vi "Generic command handler.vi"(8 "error in (no error)":errorcluster, 10 "Message in":refnum<class "GenericMessage.lvclass">, 11 "StageSPIM in":refnum<class "StageSPIM.lvclass">) -> (0 "error out":errorcluster, 2 "value":string, 3 "StageSPIM out":refnum<class "StageSPIM.lvclass">)   [LabVIEW 2012, in "StageSPIM.lvclass"]
doc: "The generic_command_handler processes the command 'generic'. Commands which are not part of the predefined list of commands fall under the 'generic' command for special activity."
uses:
  StageSPIM.lvclass
  <vilib>/Distrio/Murmex/GenericMessage/GenericMessage.lvclass
  <vilib>/Distrio/Murmex/Murmex/Murmex.lvclass
  StageSPIM.lvclass/StageSPIM.ctl
  <vilib>/Distrio/Murmex/ProceedMessage/ProceedMessage.lvclass
  <vilib>/Distrio/Murmex/Message/Message.lvclass
panel:
  # "This method is called when the GENERIC\ntrigger is sent. \n\nOverride this method when your component needs to\nrespond to this trigger. \n\nCall parent for proper implementation"
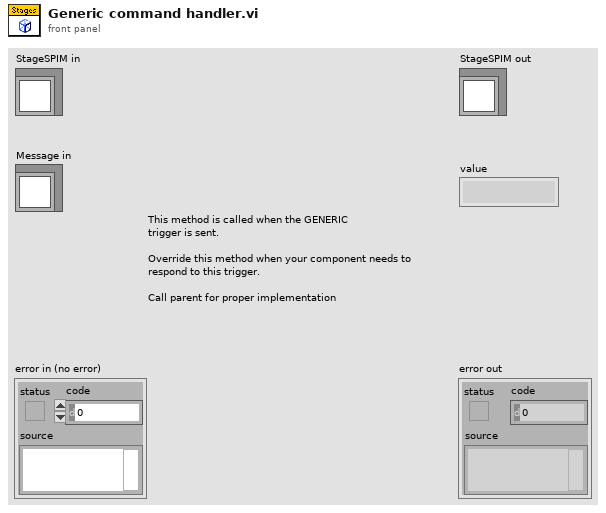
[diagram p1: front panel]
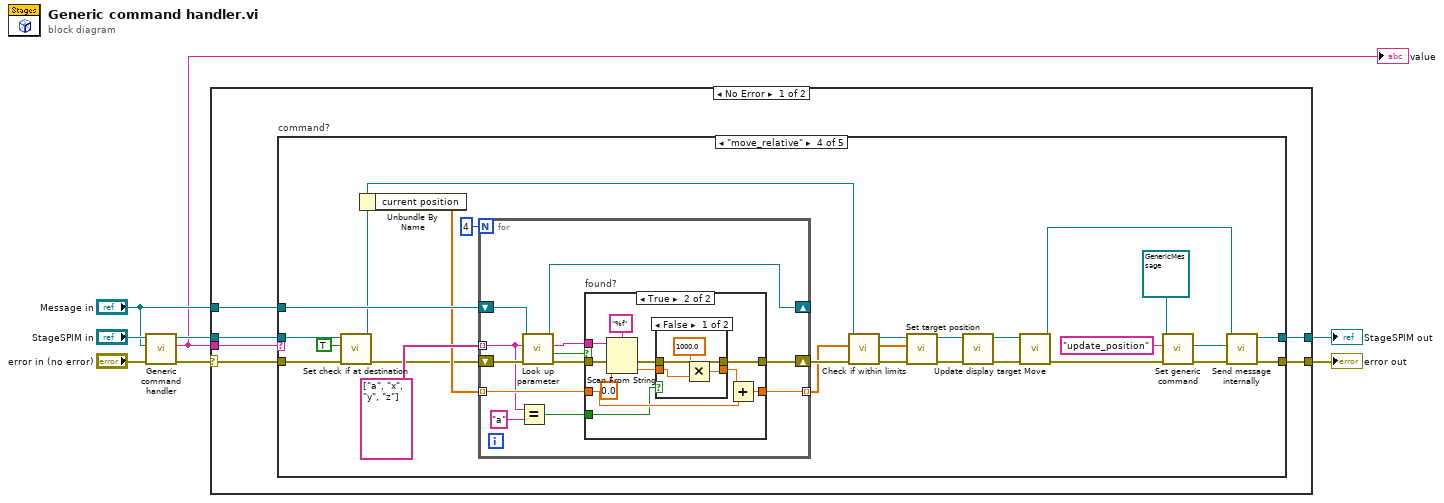
[diagram p0: block diagram]
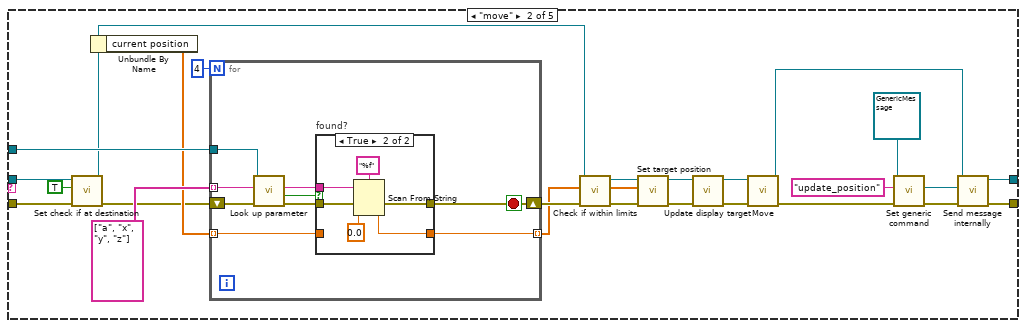
[diagram p3: hidden frame]
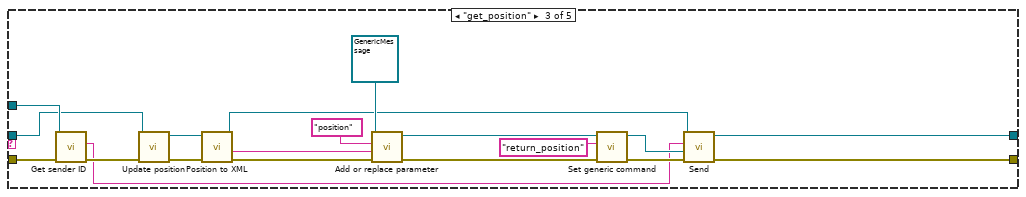
[diagram p5: hidden frame]
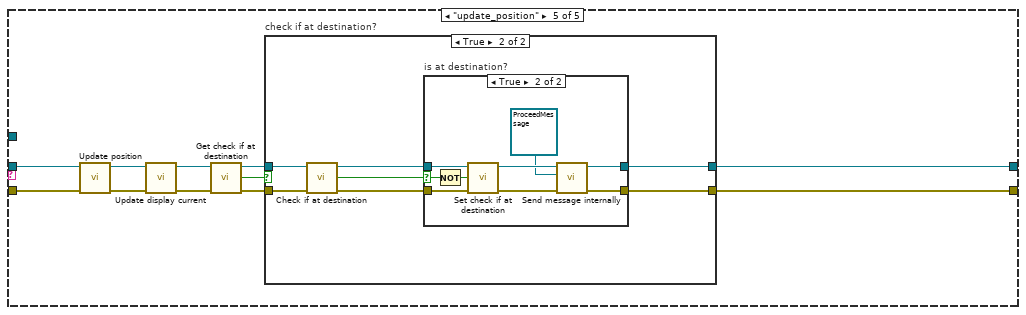
[diagram p8: hidden frame]
diagram:
  n1 = call-parent "Generic command handler.vi"("error in (no error)"="error in (no error)", "Message in"="Message in", "Murmex in"="StageSPIM in") -> ("error out"=w6:errorcluster, "value"=w3:string, "Murmex out"=w5:refnum<class "StageSPIM.lvclass">)  [unwired: 6 in]
  "value" <- w3
  n2 = case shown="No Error" w6 {
    selector: w6 -> [w13 w167]
    tunnel: w3 -> [w14 _]
    tunnel: w5 -> [w12 w168]
    tunnel: "Message in" -> [w11 _]
    tunnel: [w10 w167] -> w2
    tunnel: [w9 w168] -> w1
    frame No Error {
      n3 = case "command?" shown="\"move_relative\"" w14 {
        tunnel: w13 -> [w15 w31 w78 w93 w146]
        tunnel: w12 -> [w16 w33 w64 w95 w145]
        tunnel: w11 -> [_ w38 w77 w100 _]
        tunnel: [w15 w24 w60 w86 w140] -> w10
        tunnel: [w16 w21 w61 w83 w141] -> w9
        frame Default {
        }
        frame "move" {
          n4 = call-dynamic "Set check if at destination.vi"("error in (no error)"=w31, "check if at destination"=TRUE, "StageSPIM in"=w33) -> ("error out"=w30:errorcluster, "StageSPIM out"=w32:refnum<class "StageSPIM.lvclass">)  [unwired: 7 in]
          n5 = Unbundle By Name(w32) -> ("current position"=w35:dbl[])
          n6 = for {
            N: 4 -> [_]
            shift-right: [w43] -> w39
            shift-left: w30 -> [w51]
            tunnel: string[] ["a", "x", "y", "z"] -> [w50] mode=indexing
            tunnel: w35 -> [w45] mode=indexing
            tunnel: [w44] -> w34 mode=indexing
            tunnel: w38 -> [w46]
            stop <- w43 stop-if-true
            n7 = call <vilib>:"Look up parameter.vi"("error in (no error)"=w51, "name"=w50, "Message in"=w46) -> ("error out"=w49:errorcluster, "found?"=w48:bool, "key"=w47:string)  [unwired: 5 in, 1 out]
            n8 = case "found?" shown="True" w48 {
              tunnel: w49 -> [w53 w59]
              tunnel: [w53 w58] -> w43
              tunnel: w47 -> [_ w56]
              tunnel: [w52 w54] -> w44
              tunnel: w45 -> [w52 _]
              frame False {
              }
              frame True {
                n9 = Scan From String(format string="%f", input string=w56, error in=w59, default 1=0.0 ("default value 1")) -> (error out=w58:errorcluster, output 1=w54:dbl)  [unwired: 1 in, 2 out]
              }
            }
          }
          n10 = call-dynamic "Check if within limits.vi"("error in (no error)"=w39, "Position array in"=w34, "StageSPIM in"=w32) -> ("error out"=w41:errorcluster, "Approved postion array"=w40:dbl[], "StageSPIM out"=w42:refnum<class "StageSPIM.lvclass">)  [unwired: 4 in, 2 out]
          n11 = call-dynamic "Set target position.vi"("error in (no error)"=w41, "target position"=w40, "StageSPIM in"=w42) -> ("error out"=w20:errorcluster, "StageSPIM out"=w18:refnum<class "StageSPIM.lvclass">)  [unwired: 7 in]
          n12 = call-dynamic "Update display target.vi"("error in (no error)"=w20, "StageSPIM in"=w18) -> ("error out"=w19:errorcluster, "StageSPIM out"=w17:refnum<class "StageSPIM.lvclass">)  [unwired: 8 in]
          n13 = call-dynamic "Move.vi"("error in (no error)"=w19, "StageSPIM in"=w17) -> ("error out"=w28:errorcluster, "StageSPIM out"=w22:refnum<class "StageSPIM.lvclass">)  [unwired: 8 in]
          n14 = call <vilib>:"Set generic command.vi"("error in (no error)"=w28, "generic command"="update_position", "GenericMessage in"=refnum<class "GenericMessage.lvclass"> refnum ("Distrio Murmex 1.1:GenericMessage")) -> ("error out"=w27:errorcluster, "GenericMessage out"=w23:refnum<class "GenericMessage.lvclass">)  [unwired: 7 in]
          n15 = call <vilib>:"Send message internally.vi"("error in (no error)"=w27, "Message"=w23, "Murmex in"=w22) -> ("error out"=w24:errorcluster, "Murmex out"=w21:refnum<class "StageSPIM.lvclass">)  [unwired: 7 in]
        }
        frame "get_position" {
          n16 = call <vilib>:"Get sender ID.vi"("error in (no error)"=w78, "Message in"=w77) -> ("error out"=w76:errorcluster, "sender"=w72:string)  [unwired: 7 in, 1 out]
          n17 = call-dynamic "Update position.vi"("error in (no error)"=w76, "StageSPIM in"=w64) -> ("error out"=w66:errorcluster, "StageSPIM out"=w63:refnum<class "StageSPIM.lvclass">)  [unwired: 8 in]
          n18 = call-dynamic "Position to XML.vi"("error in (no error)"=w66, "StageSPIM in"=w63) -> ("error out"=w65:errorcluster, "XML string"=w62:string, "StageSPIM out"=w67:refnum<class "StageSPIM.lvclass">)  [unwired: 7 in]
          n19 = call <vilib>:"Add or replace parameter.vi"("error in (no error)"=w65, "value"=w62, "name"="position", "Message in"=refnum<class "GenericMessage.lvclass"> refnum ("Distrio Murmex 1.1:GenericMessage")) -> ("error out"=w70:errorcluster, "Message out"=w69:refnum<class "GenericMessage.lvclass">)  [unwired: 6 in]
          n20 = call <vilib>:"Set generic command.vi"("error in (no error)"=w70, "generic command"="return_position", "GenericMessage in"=w69) -> ("error out"=w74:errorcluster, "GenericMessage out"=w73:refnum<class "GenericMessage.lvclass">)  [unwired: 7 in]
          n21 = call <vilib>:"Send.vi"("error in (no error)"=w74, "Message"=w73, "recipient"=w72, "Murmex in"=w67) -> ("error out"=w60:errorcluster, "Murmex out"=w61:refnum<class "StageSPIM.lvclass">)  [unwired: 6 in]
        }
        frame "move_relative" {
          n22 = call-dynamic "Set check if at destination.vi"("error in (no error)"=w93, "check if at destination"=TRUE, "StageSPIM in"=w95) -> ("error out"=w92:errorcluster, "StageSPIM out"=w94:refnum<class "StageSPIM.lvclass">)  [unwired: 7 in]
          n23 = Unbundle By Name(w94) -> ("current position"=w97:dbl[])
          n24 = for {
            N: 4 -> [_]
            shift-right: [w113] -> w101
            shift-left: w92 -> [w116]
            tunnel: string[] ["a", "x", "y", "z"] -> [w107] mode=indexing
            shift-right: [w110] -> _
            shift-left: w100 -> [w111]
            tunnel: w97 -> [w109] mode=indexing
            tunnel: [w108] -> w96 mode=indexing
            n25 = Equal?(x=w107, y="a") -> (x = y?=w105:bool)
            n26 = call <vilib>:"Look up parameter.vi"("error in (no error)"=w116, "name"=w107, "Message in"=w111) -> ("error out"=w115:errorcluster, "found?"=w114:bool, "key"=w112:string, "Message out"=w110:refnum<class "GenericMessage.lvclass">)  [unwired: 5 in]
            n27 = case "found?" shown="True" w114 {
              tunnel: w115 -> [w118 w129]
              tunnel: [w118 w122] -> w113
              tunnel: w112 -> [_ w127]
              tunnel: [w117 w125] -> w108
              tunnel: w109 -> [w117 w124]
              tunnel: w105 -> [_ w123]
              frame False {
              }
              frame True {
                n28 = Scan From String(format string="%f", input string=w127, error in=w129, default 1=0.0 ("default value 1")) -> (error out=w121:errorcluster, output 1=w119:dbl)  [unwired: 1 in, 2 out]
                n29 = case shown="False" w123 {
                  tunnel: [w133 w135] -> w122
                  tunnel: w121 -> [w133 w135]
                  tunnel: [w132 w134] -> w120
                  tunnel: w119 -> [w131 w134]
                  frame False {
                    n30 = Multiply(x=1000.0, y=w131) -> (x*y=w132:dbl)
                  }
                  frame True {
                  }
                }
                n31 = Add(x=w120, y=w124) -> (x+y=w125:dbl)
              }
            }
          }
          n32 = call-dynamic "Check if within limits.vi"("error in (no error)"=w101, "Position array in"=w96, "StageSPIM in"=w94) -> ("error out"=w103:errorcluster, "Approved postion array"=w102:dbl[], "StageSPIM out"=w104:refnum<class "StageSPIM.lvclass">)  [unwired: 4 in, 2 out]
          n33 = call-dynamic "Set target position.vi"("error in (no error)"=w103, "target position"=w102, "StageSPIM in"=w104) -> ("error out"=w82:errorcluster, "StageSPIM out"=w79:refnum<class "StageSPIM.lvclass">)  [unwired: 7 in]
          n34 = call-dynamic "Update display target.vi"("error in (no error)"=w82, "StageSPIM in"=w79) -> ("error out"=w81:errorcluster, "StageSPIM out"=w80:refnum<class "StageSPIM.lvclass">)  [unwired: 8 in]
          n35 = call-dynamic "Move.vi"("error in (no error)"=w81, "StageSPIM in"=w80) -> ("error out"=w90:errorcluster, "StageSPIM out"=w84:refnum<class "StageSPIM.lvclass">)  [unwired: 8 in]
          n36 = call <vilib>:"Set generic command.vi"("error in (no error)"=w90, "generic command"="update_position", "GenericMessage in"=refnum<class "GenericMessage.lvclass"> refnum ("Distrio Murmex 1.1:GenericMessage")) -> ("error out"=w89:errorcluster, "GenericMessage out"=w85:refnum<class "GenericMessage.lvclass">)  [unwired: 7 in]
          n37 = call <vilib>:"Send message internally.vi"("error in (no error)"=w89, "Message"=w85, "Murmex in"=w84) -> ("error out"=w86:errorcluster, "Murmex out"=w83:refnum<class "StageSPIM.lvclass">)  [unwired: 7 in]
        }
        frame "update_position" {
          n38 = call-dynamic "Update position.vi"("error in (no error)"=w146, "StageSPIM in"=w145) -> ("error out"=w139:errorcluster, "StageSPIM out"=w137:refnum<class "StageSPIM.lvclass">)  [unwired: 8 in]
          n39 = call-dynamic "Update display current.vi"("error in (no error)"=w139, "StageSPIM in"=w137) -> ("error out"=w138:errorcluster, "StageSPIM out"=w136:refnum<class "StageSPIM.lvclass">)  [unwired: 8 in]
          n40 = call-dynamic "Get check if at destination.vi"("error in (no error)"=w138, "StageSPIM in"=w136) -> ("error out"=w143:errorcluster, "check if at destination"=w144:bool, "StageSPIM out"=w142:refnum<class "StageSPIM.lvclass">)  [unwired: 7 in]
          n41 = case "check if at destination?" shown="True" w144 {
            tunnel: w143 -> [w148 w155]
            tunnel: w142 -> [w147 w154]
            tunnel: [w147 w150] -> w141
            tunnel: [w148 w149] -> w140
            frame False {
            }
            frame True {
              n42 = call-dynamic "Check if at destination.vi"("error in (no error)"=w155, "StageSPIM in"=w154) -> ("error out"=w152:errorcluster, "at destination?"=w153:bool, "StageSPIM out"=w151:refnum<class "StageSPIM.lvclass">)  [unwired: 7 in]
              n43 = case "is at destination?" shown="True" w153 {
                selector: w153 -> [_ w165]
                tunnel: w152 -> [w157 w166]
                tunnel: w151 -> [w156 w163]
                tunnel: [w157 w159] -> w149
                tunnel: [w156 w158] -> w150
                frame False {
                }
                frame True {
                  n44 = Not(x=w165) -> (.not. x?=w164:bool)
                  n45 = call-dynamic "Set check if at destination.vi"("error in (no error)"=w166, "check if at destination"=w164, "StageSPIM in"=w163) -> ("error out"=w162:errorcluster, "StageSPIM out"=w161:refnum<class "StageSPIM.lvclass">)  [unwired: 7 in]
                  n46 = call <vilib>:"Send message internally.vi"("error in (no error)"=w162, "Message"=refnum<class "ProceedMessage.lvclass"> refnum ("Distrio Murmex 1.1:ProceedMessage"), "Murmex in"=w161) -> ("error out"=w159:errorcluster, "Murmex out"=w158:refnum<class "StageSPIM.lvclass">)  [unwired: 7 in]
                }
              }
            }
          }
        }
      }
    }
    frame Error {
    }
  }
  "error out" <- w2
  "StageSPIM out" <- w1
